vi "TIO RPC Test.vi"() -> ()   [LabVIEW 2022 SP3]
uses:
  <instrlib>/tio-labview/TIO Library/TIO Serial Port Name Search.vi
  <vilib>/Utility/tcp.llb/UDP Multicast Open.vi
  <vilib>/Utility/tcp.llb/UDP Multicast Read-Write Open.vi
  <instrlib>/tio-labview/TIO Library/TIO Serial Port Discovery.vi
  <vilib>/Instr/_visa.llb/VISA Configure Serial Port (Instr).vi
panel:
  in  "RPC Payload":string
  in  "RPC Named Request":string="dev.desc"
  out "error out":errorcluster
  out "RPC Reply":string
  in  "URL":refnum<visa-resource-name>="tcp://localhost"
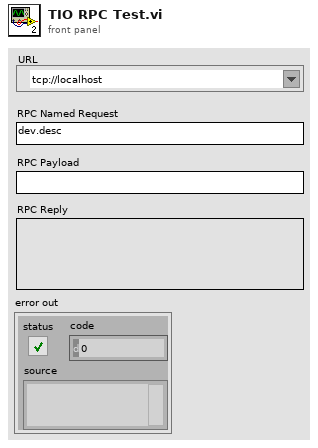
[diagram p1: front panel]
types:
  T1 = cluster{"Type":enum16{"Serial", "TCP", "UDP", "mUDP"}, "URL":refnum<visa-resource-name>, "TO":u32, "Addr":u32, "Port":i32, "TCP":refnum<k5>, "UDP":refnum<k16>, "Route":string}
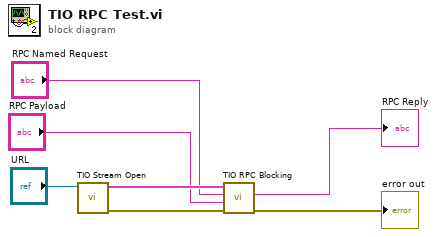
[diagram p0: block diagram]
diagram:
  n1 = call <instrlib>:"TIO Stream Open.vi"("URL"="URL") -> ("error out"=w6:errorcluster, "TC Connection"=w5:T1)  [unwired: 8 in, 1 out]
  n2 = call <instrlib>:"TIO RPC Blocking.vi"("error in (no error)"=w6, "Payload"="RPC Payload", "Named Method"="RPC Named Request", "TC Connection"=w5) -> ("error out"=→"error out":errorcluster, "Respose"=→"RPC Reply":string)  [unwired: 4 in, 2 out]
